vi "Start Sync.vi"(8 "error in (no error)":errorcluster, 10 "current time":timestamp, 11 "gRPC Server in":refnum<class "HVC5.lvclass">) -> (0 "error out":errorcluster, 3 "gRPC Server out":refnum<class "HVC5.lvclass">)   [LabVIEW 2019, in "HVC5.lvlib" / "HVC5.lvclass"]
uses:
  HVC5.lvclass
  RPC Messages/measurementservice_DMMConfigResponse/measurementservice_DMMConfigResponse_Data.ctl
  RPC Messages/measurementservice_ErrorOut/measurementservice_ErrorOut_Data.ctl
  RPC Messages/measurementservice_SMUConfigResponse/measurementservice_SMUConfigResponse_Data.ctl
  HVC5.lvclass/HVC5.ctl
  RPC Messages/measurementservice_QueryResponse/measurementservice_QueryResponse_Data.ctl
  RPC Messages/measurementservice_DMMOpenSessionResponse/measurementservice_DMMOpenSessionResponse_Data.ctl
  RPC Messages/measurementservice_DMMVoltageData/measurementservice_DMMVoltageData_Data.ctl
  RPC Messages/measurementservice_DMMCloseSessionResponse/measurementservice_DMMCloseSessionResponse_Data.ctl
  RPC Messages/measurementservice_DMMSelfCalResponse/measurementservice_DMMSelfCalResponse_Data.ctl
  RPC Messages/measurementservice_DMMResetResponse/measurementservice_DMMResetResponse_Data.ctl
  RPC Messages/measurementservice_SMUOpenSessionResponse/measurementservice_SMUOpenSessionResponse_Data.ctl
  RPC Messages/measurementservice_SMUCurrentData/measurementservice_SMUCurrentData_Data.ctl
  RPC Messages/measurementservice_SMUDisableResponse/measurementservice_SMUDisableResponse_Data.ctl
  RPC Messages/measurementservice_SMUEnableResponse/measurementservice_SMUEnableResponse_Data.ctl
  RPC Messages/measurementservice_SMUCloseSessionResponse/measurementservice_SMUCloseSessionResponse_Data.ctl
  RPC Messages/measurementservice_SMUSelfCalResponse/measurementservice_SMUSelfCalResponse_Data.ctl
  RPC Messages/measurementservice_SMUResetResponse/measurementservice_SMUResetResponse_Data.ctl
  RPC Messages/measurementservice_NI2576MUXOpenSessionResponse/measurementservice_NI2576MUXOpenSessionResponse_Data.ctl
  RPC Messages/measurementservice_NI2576MUXCloseSessionResponse/measurementservice_NI2576MUXCloseSessionResponse_Data.ctl
  RPC Messages/measurementservice_NI2576MUXDisconnectAllResponse/measurementservice_NI2576MUXDisconnectAllResponse_Data.ctl
  <instrlib>/niSwitch/niSwitch.llb/niSwitch Connect Channels (Single).vi
  RPC Messages/measurementservice_NI2576MUXCloseChannelResponse/measurementservice_NI2576MUXCloseChannelResponse_Data.ctl
  <instrlib>/niSwitch/niSwitch.llb/niSwitch Disconnect Channels (Single).vi
  RPC Messages/measurementservice_NI2576MUXOpenChannelResponse/measurementservice_NI2576MUXOpenChannelResponse_Data.ctl
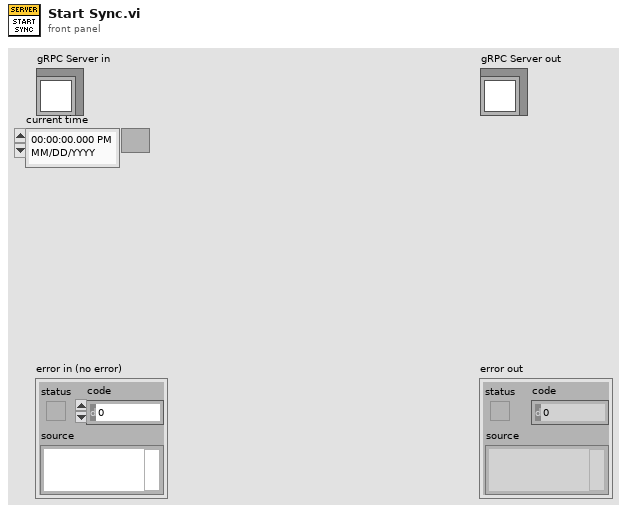
[diagram p1: front panel]
types:
  T1 = typedef "HVC5.lvlib/HVC5.lvclass/measurementservice_DMMConfigResponse_Data.ctl" = cluster{"DMMFunction":i32, "DMMResolution":sgl, "DMMRange":sgl, "DMMSampleCount":i32, "DMMApertureTimeUnit":i32, "DMMApertureTime":sgl, "DMMNumberofAverages":i32, "DMMAutoZero":i32, "DMMADCCalibration":i32, "DMMSettleTime":sgl, "error":T2}
  T2 = typedef "HVC5.lvlib/HVC5.lvclass/measurementservice_ErrorOut_Data.ctl" = cluster{"errCode":i32, "errMessage":string}
  T3 = typedef "HVC5.lvlib/HVC5.lvclass/measurementservice_SMUConfigResponse_Data.ctl" = cluster{"SMUChannels":string, "SMUSourceMode":i32, "SMUOutputFunction":i32, "SMUSourceTransientResponse":i32, "SMUCurrent":sgl, "SMUCurrentLevelRange":sgl, "SMUMeasurementSense":i32, "SMUApertureTimeUnit":i32, "SMUMeasurementApertureTime":sgl, "SMUSourceAdvancedSourceDelay":sgl, "SMUVoltage":sgl, "SMUMeasurementAdvancedDCNoiseRejection":i32, "error":T2}
  T4 = cluster{"DMMSession":refnum<k15>, "measurementservice_DMMConfigResponse_Data":T1, "SMUSession":refnum<k15>, "measurementservice_SMUConfigResponse_Data":T3, "NI2576Session":refnum<k15>}
  T5 = typedef "HVC5.lvlib/HVC5.lvclass/measurementservice_QueryResponse_Data.ctl" = cluster{"message":string, "status":i32}
  T6 = typedef "HVC5.lvlib/HVC5.lvclass/measurementservice_DMMOpenSessionResponse_Data.ctl" = cluster{"error":T2}
  T7 = typedef "HVC5.lvlib/HVC5.lvclass/measurementservice_DMMVoltageData_Data.ctl" = cluster{"voltage":sgl[], "error":T2}
  T8 = typedef "HVC5.lvlib/HVC5.lvclass/measurementservice_DMMCloseSessionResponse_Data.ctl" = cluster{"error":T2}
  T9 = typedef "HVC5.lvlib/HVC5.lvclass/measurementservice_DMMSelfCalResponse_Data.ctl" = cluster{"error":T2}
  T10 = typedef "HVC5.lvlib/HVC5.lvclass/measurementservice_DMMResetResponse_Data.ctl" = cluster{"error":T2}
  T11 = typedef "HVC5.lvlib/HVC5.lvclass/measurementservice_SMUOpenSessionResponse_Data.ctl" = cluster{"error":T2}
  T12 = typedef "HVC5.lvlib/HVC5.lvclass/measurementservice_SMUCurrentData_Data.ctl" = cluster{"current":sgl, "error":T2}
  T13 = typedef "HVC5.lvlib/HVC5.lvclass/measurementservice_SMUDisableResponse_Data.ctl" = cluster{"error":T2}
  T14 = typedef "HVC5.lvlib/HVC5.lvclass/measurementservice_SMUEnableResponse_Data.ctl" = cluster{"error":T2}
  T15 = typedef "HVC5.lvlib/HVC5.lvclass/measurementservice_SMUCloseSessionResponse_Data.ctl" = cluster{"error":T2}
  T16 = typedef "HVC5.lvlib/HVC5.lvclass/measurementservice_SMUSelfCalResponse_Data.ctl" = cluster{"error":T2}
  T17 = typedef "HVC5.lvlib/HVC5.lvclass/measurementservice_SMUResetResponse_Data.ctl" = cluster{"error":T2}
  T18 = typedef "HVC5.lvlib/HVC5.lvclass/measurementservice_NI2576MUXOpenSessionResponse_Data.ctl" = cluster{"error":T2}
  T19 = typedef "HVC5.lvlib/HVC5.lvclass/measurementservice_NI2576MUXCloseChannelResponse_Data.ctl" = cluster{"error":T2}
  T20 = typedef "HVC5.lvlib/HVC5.lvclass/measurementservice_NI2576MUXOpenChannelResponse_Data.ctl" = cluster{"error":T2}
  T21 = typedef "HVC5.lvlib/HVC5.lvclass/measurementservice_NI2576MUXDisconnectAllResponse_Data.ctl" = cluster{"error":T2}
  T22 = typedef "HVC5.lvlib/HVC5.lvclass/measurementservice_NI2576MUXCloseSessionResponse_Data.ctl" = cluster{"error":T2}
  T23 = typedef "HVC5.lvlib/HVC5.lvclass/Server gRPC UEs.ctl" = cluster{"Invoke gRPC UE":refnum<user-event>, "Query gRPC UE":refnum<user-event>, "Register gRPC UE":refnum<user-event>, "OpenDMMSession gRPC UE":refnum<user-event>, "ConfigureDMM gRPC UE":refnum<user-event>, "PerformDMMVoltageMeasurement gRPC UE":refnum<user-event>, "CloseDMMSession gRPC UE":refnum<user-event>, "SelfCalibrateDMM gRPC UE":refnum<user-event>, "ResetDMM gRPC UE":refnum<user-event>, "OpenSMUSession gRPC UE":refnum<user-event>, "ConfigureSMU gRPC UE":refnum<user-event>, "EnableSMUOutput gRPC UE":refnum<user-event>, "DisableSMUOutput gRPC UE":refnum<user-event>, "PerformSMUCurrentMeasurement gRPC UE":refnum<user-event>, "CloseSMUSession gRPC UE":refnum<user-event>, "SelfCalibrateSMU gRPC UE":refnum<user-event>, "ResetSMU gRPC UE":refnum<user-event>, "OpenNI2576MUXSession gRPC UE":refnum<user-event>, "CloseNI2576MUXChannel gRPC UE":refnum<user-event>, "OpenNI2576MUXChannel gRPC UE":refnum<user-event>, "DisconnectAllNI2576MUXChannels gRPC UE":refnum<user-event>, "CloseNI2576MUXSession gRPC UE":refnum<user-event>, "ResetNI2576MUX gRPC UE":refnum<user-event>}
  T24 = typedef "HVC5.lvlib/gprc-lvsupport.lvlib/grpcId.ctl" = u64
  T25 = typedef "HVC5.lvlib/HVC5.lvclass/measurementservice_QueryRequest_Data.ctl" = cluster{"query":string}
  T26 = typedef "HVC5.lvlib/HVC5.lvclass/measurementservice_DMMOpenSessionRequest_Data.ctl" = cluster{"DMMName":string}
  T27 = typedef "HVC5.lvlib/HVC5.lvclass/measurementservice_DMMConfigRequest_Data.ctl" = cluster{"DMMFunction":i32, "DMMResolution":sgl, "DMMRange":sgl, "DMMSampleCount":i32, "DMMApertureTimeUnit":i32, "DMMApertureTime":sgl, "DMMNumberofAverages":i32, "DMMAutoZero":i32, "DMMADCCalibration":i32, "DMMSettleTime":sgl}
  T28 = typedef "HVC5.lvlib/HVC5.lvclass/measurementservice_SMUOpenSessionRequest_Data.ctl" = cluster{"SMUName":string}
  T29 = typedef "HVC5.lvlib/HVC5.lvclass/measurementservice_SMUConfigRequest_Data.ctl" = cluster{"SMUChannels":string, "SMUSourceMode":i32, "SMUOutputFunction":i32, "SMUSourceTransientResponse":i32, "SMUCurrent":sgl, "SMUCurrentLevelRange":sgl, "SMUMeasurementSense":i32, "SMUApertureTimeUnit":i32, "SMUMeasurementApertureTime":sgl, "SMUSourceAdvancedSourceDelay":sgl, "SMUVoltage":sgl, "SMUMeasurementAdvancedDCNoiseRejection":i32}
  T30 = typedef "HVC5.lvlib/HVC5.lvclass/measurementservice_NI2576MUXOpenSessionRequest_Data.ctl" = cluster{"NI2576MUXName":string, "NI2576MUXTopology":string}
  T31 = typedef "HVC5.lvlib/HVC5.lvclass/measurementservice_NI2576MUXCloseChannelRequest_Data.ctl" = cluster{"Channel1":string, "Channel2":string}
  T32 = typedef "HVC5.lvlib/HVC5.lvclass/measurementservice_NI2576MUXOpenChannelRequest_Data.ctl" = cluster{"Channel1":string, "Channel2":string}
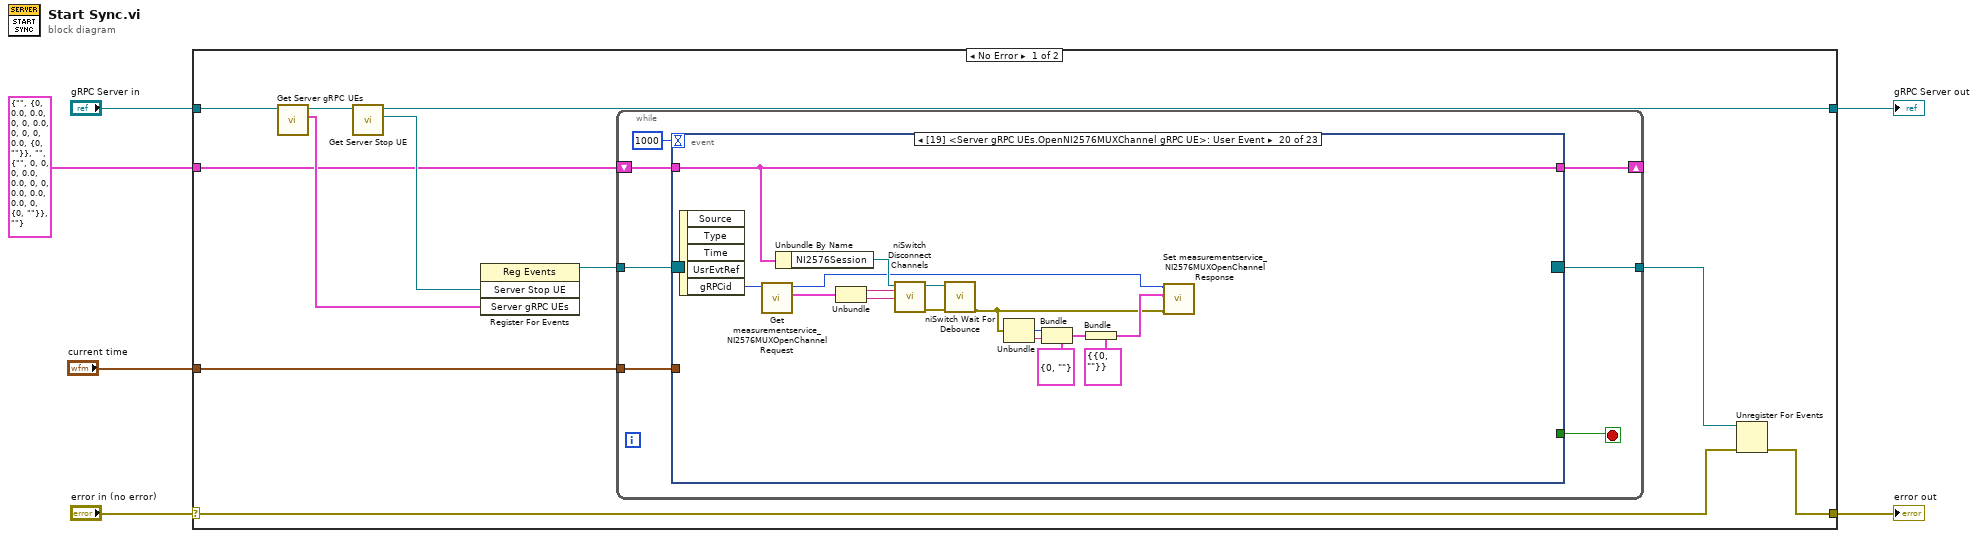
[diagram p0: block diagram]
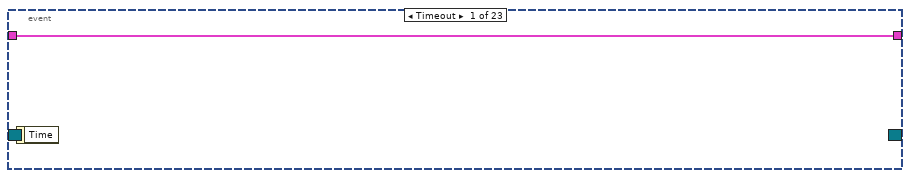
[diagram p2: hidden frame]
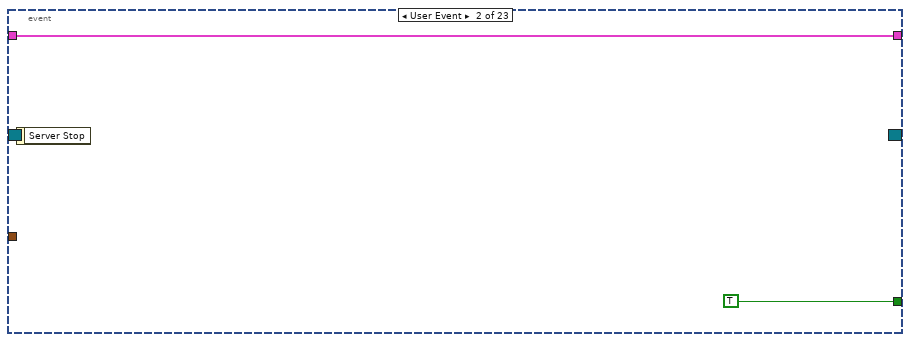
[diagram p3: hidden frame]
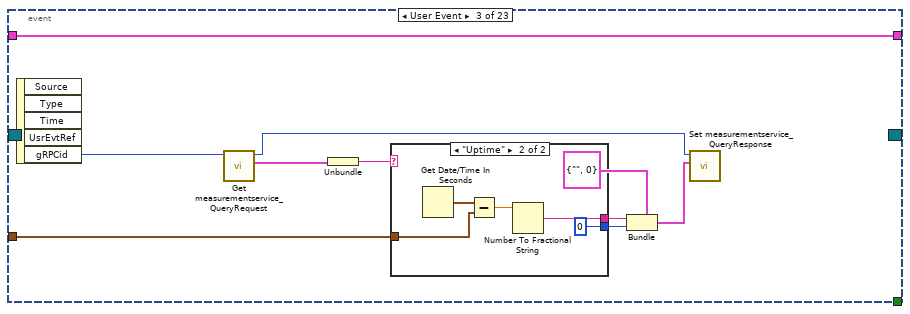
[diagram p4: hidden frame]
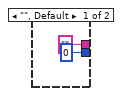
[diagram p5: hidden frame]
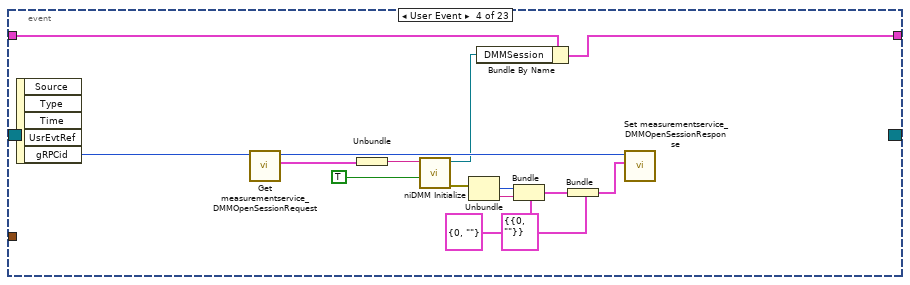
[diagram p6: hidden frame]
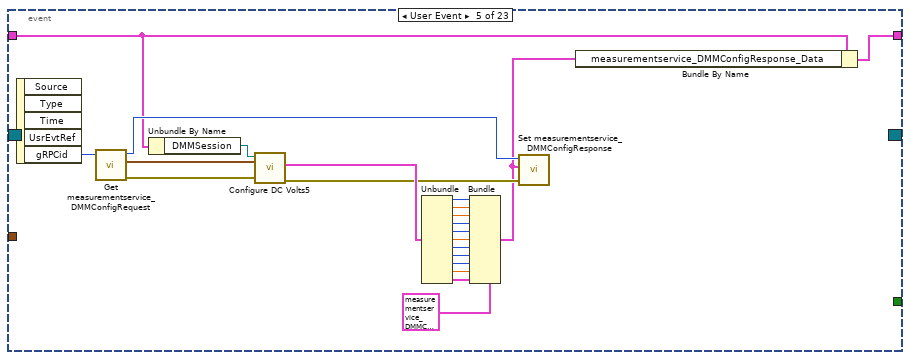
[diagram p7: hidden frame]
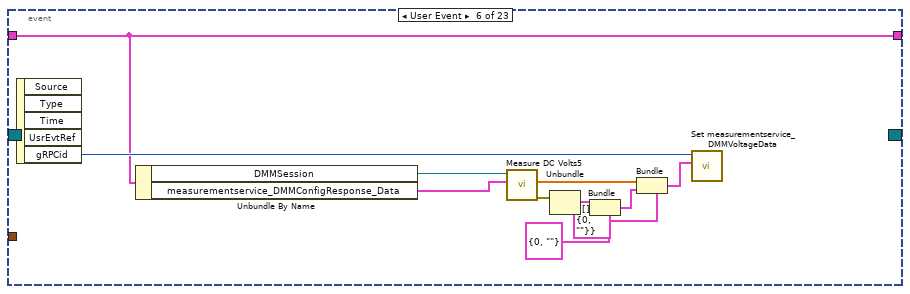
[diagram p8: hidden frame]
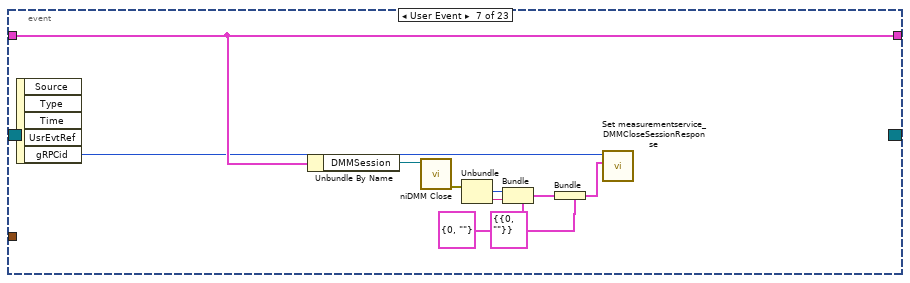
[diagram p9: hidden frame]
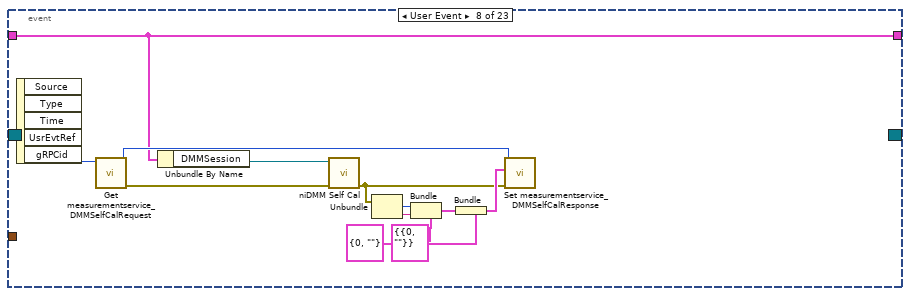
[diagram p10: hidden frame]
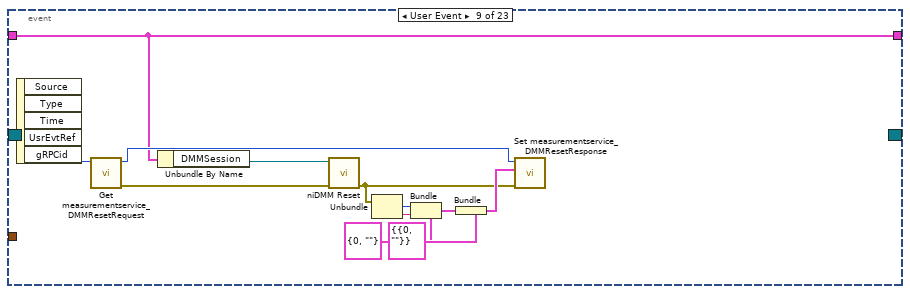
[diagram p11: hidden frame]
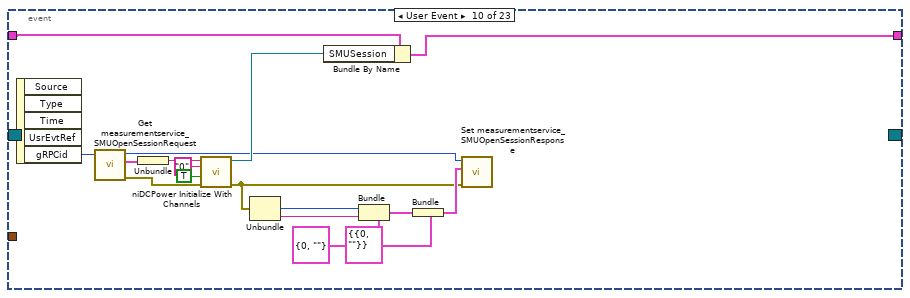
[diagram p12: hidden frame]
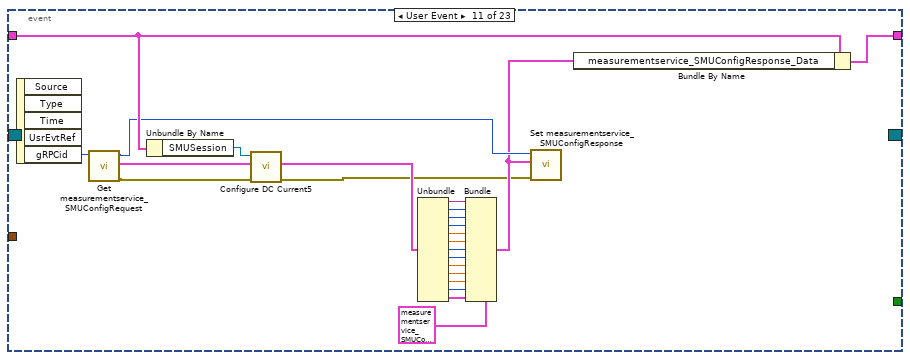
[diagram p13: hidden frame]
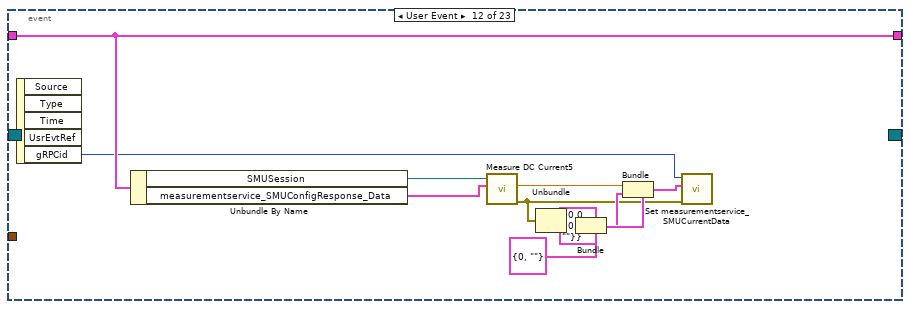
[diagram p14: hidden frame]
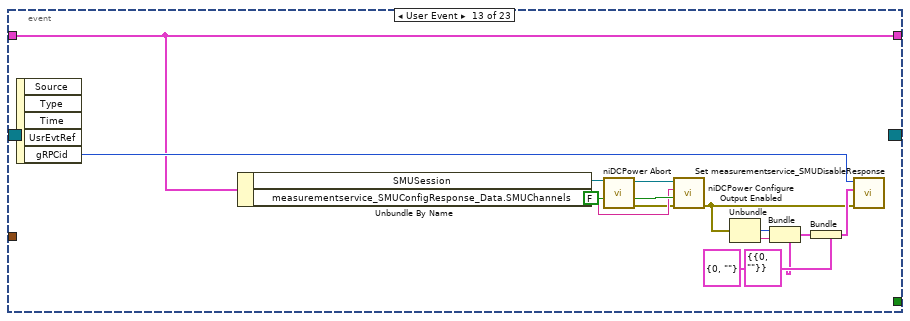
[diagram p15: hidden frame]
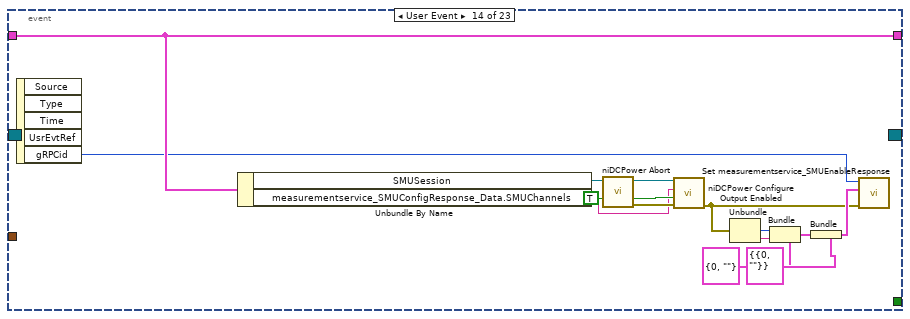
[diagram p16: hidden frame]
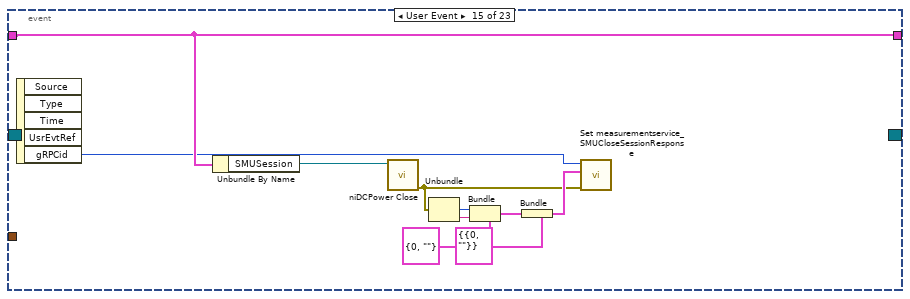
[diagram p17: hidden frame]
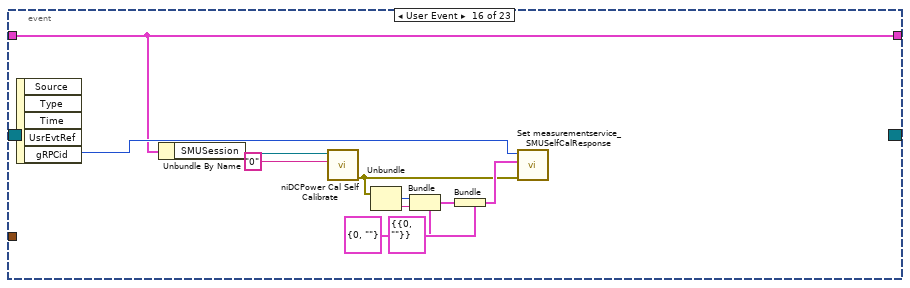
[diagram p18: hidden frame]
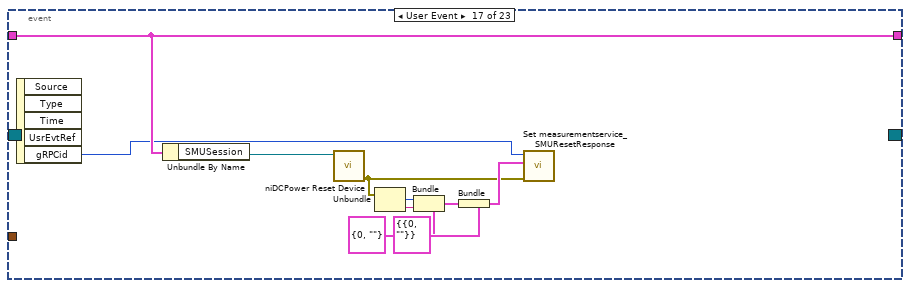
[diagram p19: hidden frame]
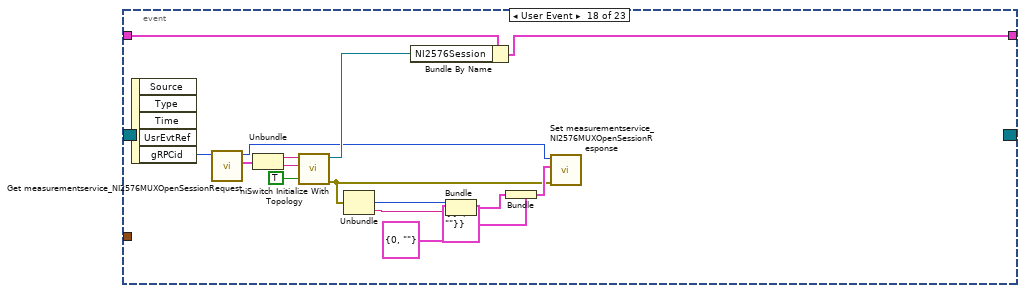
[diagram p20: hidden frame]
diagram:
  n1 = case shown="No Error" "error in (no error)" {
    selector: "error in (no error)" -> [w10 w318]
    tunnel: [w9 w318] -> w5
    tunnel: [w13 w317] -> w3
    tunnel: "gRPC Server in" -> [w17 w317]
    tunnel: "current time" -> [w8 _]
    tunnel: T4 {"DMMSession"="", "measurementservice_DMMConfigResponse_Data"={"DMMFunction"=0, "DMMResolution"=0.0, "DMMRange"=0.0, "DMMSampleCount"=0, "DMMApertureTimeUnit"=0, "DMMApertureTime"=0.0, "DMMNumberofAverages"=0, "DMMAutoZero"=0, "DMMADCCalibration"=0, "DMMSettleTime"=0.0, "error"={"errCode"=0, "errMessage"=""}}, "SMUSession"="", "measurementservice_SMUConfigResponse_Data"={"SMUChannels"="", "SMUSourceMode"=0, "SMUOutputFunction"=0, "SMUSourceTransientResponse"=0, "SMUCurrent"=0.0, "SMUCurrentLevelRange"=0.0, "SMUMeasurementSense"=0, "SMUApertureTimeUnit"=0, "SMUMeasurementApertureTime"=0.0, "SMUSourceAdvancedSourceDelay"=0.0, "SMUVoltage"=0.0, "SMUMeasurementAdvancedDCNoiseRejection"=0, "error"={"errCode"=0, "errMessage"=""}}, "NI2576Session"=""} -> [w7 _]
    frame No Error {
      n2 = call "Get Server gRPC UEs.vi"("OOP Server in"=w17) -> ("Server gRPC UEs"=w14:T23, "OOP Server out"=w16:refnum<class "HVC5.lvclass">)  [unwired: 9 in]
      n3 = call "Get Server Stop UE.vi"("OOP Server in"=w16) -> ("Server Stop UE"=w15:refnum<user-event>, "OOP Server out"=w13:refnum<class "HVC5.lvclass">)  [unwired: 9 in]
      n4 = register-events(w15, w14) -> (reference out=w12:refnum<event-registration>)  [unwired: 2 in, 1 out]
      n5 = while {
        tunnel: w12 -> [w24]
        tunnel: [w22] -> w11
        tunnel: w8 -> [w20]
        shift-right: [w18] -> _
        shift-left: w7 -> [w19]
        stop <- w23 stop-if-true
        n6 = event "RPC Methods Event Structure" shown="[19] <Server gRPC UEs.OpenNI2576MUXChannel gRPC UE>: User Event" {
          selector: w24 -> [_ _ _ _ _ _ _ _ _ _ _ _ _ _ _ _ _ _ _ _ _ _ _]
          dyn-events: [_ _ _ _ _ _ _ _ _ _ _ _ _ _ _ _ _ _ _ _ _ _ _] -> w22
          timeout: 1000 -> [_ _ _ _ _ _ _ _ _ _ _ _ _ _ _ _ _ _ _ _ _ _ _]
          tunnel: [_ TRUE _ _ _ _ _ _ _ _ _ _ _ _ _ _ _ _ _ _ _ _ _] -> w23
          tunnel: w20 -> [_ _ w35 _ _ _ _ _ _ _ _ _ _ _ _ _ _ _ _ _ _ _ _]
          tunnel: w19 -> [w25 w26 w28 w47 w62 w82 w96 w104 w116 w137 w157 w178 w185 w205 w215 w219 w237 w250 w264 w282 w288 w298 w308]
          tunnel: [w25 w26 w28 w45 w60 w82 w96 w104 w116 w136 w156 w178 w185 w205 w215 w219 w237 w248 w264 w282 w288 w298 w308] -> w18
          event Timeout {
            n7 = event-data() -> ()  [unwired: 1 in, 1 out]
          }
          event User Event {
            n8 = event-data() -> ()  [unwired: 1 in, 1 out]
          }
          event User Event {
            n9 = event-data() -> ("gRPCid"=w37:T24)  [unwired: 1 in, 4 out]
            n10 = call "Get measurementservice_QueryRequest.vi"("gRPCid"=w37) -> ("Message Data"=w36:T25, "gRPCid out"=w30:T24)  [unwired: 8 in, 1 out]
            n11 = Unbundle(w36) -> ("query"=w34:string)
            n12 = case shown="\"Uptime\"" w34 {
              tunnel: w35 -> [_ w43]
              tunnel: ["" w41] -> w32
              tunnel: [0 ("status") 0 ("status")] -> w31
              frame "", Default {
              }
              frame "Uptime" {
                n13 = Get Date/Time In Seconds() -> (seconds since 1Jan1904=w44:timestamp)
                n14 = Subtract(x=w44, y=w43) -> (x-y=w42:dbl)
                n15 = Number To Fractional String(number=w42) -> (F-format string=w41:string)  [unwired: 3 in]
              }
            }
            n16 = Bundle(cluster=T5 {"message"="", "status"=0} ("measurementservice_QueryResponse_Data"), "message"=w32, "status"=w31) -> (w29:T5)
            n17 = call "Set measurementservice_QueryResponse.vi"("Message Data"=w29, "gRPCid"=w30) -> ()  [unwired: 9 in, 1 out]
          }
          event User Event {
            n18 = event-data() -> ("gRPCid"=w59:T24)  [unwired: 1 in, 4 out]
            n19 = call "Get measurementservice_DMMOpenSessionRequest.vi"("gRPCid"=w59) -> ("Message Data"=w58:T26, "gRPCid out"=w48:T24)  [unwired: 8 in, 1 out]
            n20 = Unbundle(w58) -> ("DMMName"=w57:string)
            n21 = call <instrlib>:"niDMM Initialize.vi"("Reset"=TRUE, "Instrument Descriptor"=w57) -> ("error out"=w55:errorcluster, "instrument handle out"=w46:refnum<k15>)  [unwired: 8 in]
            n22 = Unbundle(w55) -> ("code"=w52:i32, "source"=w51:string)  [unwired: 1 out]
            n23 = Bundle By Name(cluster=w47, "DMMSession"=w46) -> (w45:T4)
            n24 = Bundle(cluster=T2 {"errCode"=0, "errMessage"=""} ("error"), "errCode"=w52, "errMessage"=w51) -> (w50:T2)
            n25 = Bundle(cluster=T6 {"error"={"errCode"=0, "errMessage"=""}} ("measurementservice_DMMOpenSessionResponse_Data"), "error"=w50) -> (w49:T6)
            n26 = call "Set measurementservice_DMMOpenSessionResponse.vi"("Message Data"=w49, "gRPCid"=w48) -> ()  [unwired: 9 in, 1 out]
          }
          event User Event {
            n27 = event-data() -> ("gRPCid"=w81:T24)  [unwired: 1 in, 4 out]
            n28 = call "Get measurementservice_DMMConfigRequest.vi"("gRPCid"=w81) -> ("error out"=w65:errorcluster, "Message Data"=w80:T27, "gRPCid out"=w77:T24)  [unwired: 8 in]
            n29 = Unbundle By Name(w62) -> ("DMMSession"=w79:refnum<k15>)
            n30 = call "Configure DC Volts5.vi"("error in (no error)"=w65, "measurementservice_DMMConfigRequest_Data"=w80, "DMMSession"=w79) -> ("error out"=w63:errorcluster, "measurementservice_DMMConfigResponse_Data"=w76:T1)  [unwired: 7 in]
            n31 = Unbundle(w76) -> ("DMMFunction"=w75:i32, "DMMResolution"=w74:sgl, "DMMRange"=w73:sgl, "DMMSampleCount"=w72:i32, "DMMApertureTimeUnit"=w71:i32, "DMMApertureTime"=w70:sgl, "DMMNumberofAverages"=w69:i32, "DMMAutoZero"=w68:i32, "DMMADCCalibration"=w67:i32, "DMMSettleTime"=w66:sgl, "error"=w64:T2)
            n32 = Bundle(cluster=T1 {"DMMFunction"=0, "DMMResolution"=0.0, "DMMRange"=0.0, "DMMSampleCount"=0, "DMMApertureTimeUnit"=0, "DMMApertureTime"=0.0, "DMMNumberofAverages"=0, "DMMAutoZero"=0, "DMMADCCalibration"=0, "DMMSettleTime"=0.0, "error"={"errCode"=0, "errMessage"=""}} ("measurementservice_DMMConfigResponse_Data"), "DMMFunction"=w75, "DMMResolution"=w74, "DMMRange"=w73, "DMMSampleCount"=w72, "DMMApertureTimeUnit"=w71, "DMMApertureTime"=w70, "DMMNumberofAverages"=w69, "DMMAutoZero"=w68, "DMMADCCalibration"=w67, "DMMSettleTime"=w66, "error"=w64) -> (w61:T1)
            n33 = call "Set measurementservice_DMMConfigResponse.vi"("error in (no error)"=w63, "Message Data"=w61, "gRPCid"=w77) -> ()  [unwired: 8 in, 1 out]
            n34 = Bundle By Name(cluster=w62, "measurementservice_DMMConfigResponse_Data"=w61) -> (w60:T4)
          }
          event User Event {
            n35 = event-data() -> ("gRPCid"=w83:T24)  [unwired: 1 in, 4 out]
            n36 = Unbundle By Name(w82) -> ("DMMSession"=w93:refnum<k15>, "measurementservice_DMMConfigResponse_Data"=w92:T1)
            n37 = call "Measure DC Volts5.vi"("measurementservice_DMMConfigResponse_Data"=w92, "DMMSession"=w93) -> ("error out"=w88:errorcluster, "Measurement Array (Volts)"=w90:sgl[])  [unwired: 8 in]
            n38 = Unbundle(w88) -> ("code"=w87:i32, "source"=w86:string)  [unwired: 1 out]
            n39 = Bundle(cluster=T2 {"errCode"=0, "errMessage"=""} ("error"), "errCode"=w87, "errMessage"=w86) -> (w85:T2)
            n40 = Bundle(cluster=T7 {"voltage"=[], "error"={"errCode"=0, "errMessage"=""}} ("Message Data"), "voltage"=w90, "error"=w85) -> (w84:T7)
            n41 = call "Set measurementservice_DMMVoltageData.vi"("Message Data"=w84, "gRPCid"=w83) -> ()  [unwired: 9 in, 1 out]
          }
          event User Event {
            n42 = event-data() -> ("gRPCid"=w94:T24)  [unwired: 1 in, 4 out]
            n43 = Unbundle By Name(w96) -> ("DMMSession"=w95:refnum<k15>)
            n44 = call <instrlib>:"niDMM Close.vi"("instrument handle"=w95) -> ("error out"=w103:errorcluster)  [unwired: 10 in]
            n45 = Unbundle(w103) -> ("code"=w99:i32, "source"=w98:string)  [unwired: 1 out]
            n46 = Bundle(cluster=T2 {"errCode"=0, "errMessage"=""} ("error"), "errCode"=w99, "errMessage"=w98) -> (w97:T2)
            n47 = Bundle(cluster=T8 {"error"={"errCode"=0, "errMessage"=""}} ("measurementservice_DMMCloseSessionResponse_Data"), "error"=w97) -> (w101:T8)
            n48 = call "Set measurementservice_DMMCloseSessionResponse.vi"("Message Data"=w101, "gRPCid"=w94) -> ()  [unwired: 9 in, 1 out]
          }
          event User Event {
            n49 = event-data() -> ("gRPCid"=w115:T24)  [unwired: 1 in, 4 out]
            n50 = call "Get measurementservice_DMMSelfCalRequest.vi"("gRPCid"=w115) -> ("error out"=w106:errorcluster, "gRPCid out"=w108:T24)  [unwired: 8 in, 1 out]
            n51 = Unbundle By Name(w104) -> ("DMMSession"=w105:refnum<k15>)
            n52 = call <instrlib>:"niDMM Self Cal.vi"("error in (no error)"=w106, "instrument handle"=w105) -> ("error out"=w107:errorcluster)  [unwired: 8 in, 1 out]
            n53 = Unbundle(w107) -> ("code"=w110:i32, "source"=w109:string)  [unwired: 1 out]
            n54 = Bundle(cluster=T2 {"errCode"=0, "errMessage"=""} ("error"), "errCode"=w110, "errMessage"=w109) -> (w111:T2)
            n55 = Bundle(cluster=T9 {"error"={"errCode"=0, "errMessage"=""}} ("measurementservice_DMMSelfCalResponse_Data"), "error"=w111) -> (w113:T9)
            n56 = call "Set measurementservice_DMMSelfCalResponse.vi"("error in (no error)"=w107, "Message Data"=w113, "gRPCid"=w108) -> ()  [unwired: 8 in, 1 out]
          }
          event User Event {
            n57 = event-data() -> ("gRPCid"=w124:T24)  [unwired: 1 in, 4 out]
            n58 = call "Get measurementservice_DMMResetRequest.vi"("gRPCid"=w124) -> ("error out"=w123:errorcluster, "gRPCid out"=w120:T24)  [unwired: 8 in, 1 out]
            n59 = Unbundle By Name(w116) -> ("DMMSession"=w125:refnum<k15>)
            n60 = call <instrlib>:"niDMM Reset.vi"("error in (no error)"=w123, "instrument handle"=w125) -> ("error out"=w119:errorcluster)  [unwired: 8 in, 1 out]
            n61 = Unbundle(w119) -> ("code"=w127:i32, "source"=w126:string)  [unwired: 1 out]
            n62 = Bundle(cluster=T2 {"errCode"=0, "errMessage"=""} ("error"), "errCode"=w127, "errMessage"=w126) -> (w117:T2)
            n63 = Bundle(cluster=T10 {"error"={"errCode"=0, "errMessage"=""}} ("measurementservice_DMMResetResponse_Data"), "error"=w117) -> (w121:T10)
            n64 = call "Set measurementservice_DMMResetResponse.vi"("error in (no error)"=w119, "Message Data"=w121, "gRPCid"=w120) -> ()  [unwired: 8 in, 1 out]
          }
          event User Event {
            n65 = event-data() -> ("gRPCid"=w139:T24)  [unwired: 1 in, 4 out]
            n66 = call "Get measurementservice_SMUOpenSessionRequest.vi"("gRPCid"=w139) -> ("error out"=w130:errorcluster, "Message Data"=w138:T28, "gRPCid out"=w135:T24)  [unwired: 8 in]
            n67 = Unbundle(w138) -> ("SMUName"=w144:string)
            n68 = call <instrlib>:"niDCPower Initialize With Channels.vi"("error in (no error)"=w130, "reset (false)"=TRUE ("Reset"), "channels"="0", "resource name"=w144) -> ("error out"=w129:errorcluster, "instrument handle out"=w140:refnum<k15>)  [unwired: 6 in]
            n69 = Unbundle(w129) -> ("code"=w142:i32, "source"=w141:string)  [unwired: 1 out]
            n70 = Bundle By Name(cluster=w137, "SMUSession"=w140) -> (w136:T4)
            n71 = Bundle(cluster=T2 {"errCode"=0, "errMessage"=""} ("error"), "errCode"=w142, "errMessage"=w141) -> (w131:T2)
            n72 = Bundle(cluster=T11 {"error"={"errCode"=0, "errMessage"=""}} ("measurementservice_SMUOpenSessionResponse_Data"), "error"=w131) -> (w134:T11)
            n73 = call "Set measurementservice_SMUOpenSessionResponse.vi"("error in (no error)"=w129, "Message Data"=w134, "gRPCid"=w135) -> ()  [unwired: 8 in, 1 out]
          }
          event User Event {
            n74 = event-data() -> ("gRPCid"=w155:T24)  [unwired: 1 in, 4 out]
            n75 = call "Get measurementservice_SMUConfigRequest.vi"("gRPCid"=w155) -> ("error out"=w154:errorcluster, "Message Data"=w152:T29, "gRPCid out"=w150:T24)  [unwired: 8 in]
            n76 = Unbundle By Name(w157) -> ("SMUSession"=w153:refnum<k15>)
            n77 = call "Configure DC Current5.vi"("error in (no error)"=w154, "measurementservice_SMUConfigRequest_Data"=w152, "SMUSession"=w153) -> ("error out"=w145:errorcluster, "measurementservice_SMUConfigResponse_Data"=w151:T3)  [unwired: 7 in]
            n78 = Unbundle(w151) -> ("SMUChannels"=w168:string, "SMUSourceMode"=w167:i32, "SMUOutputFunction"=w166:i32, "SMUSourceTransientResponse"=w165:i32, "SMUCurrent"=w164:sgl, "SMUCurrentLevelRange"=w163:sgl, "SMUMeasurementSense"=w162:i32, "SMUApertureTimeUnit"=w161:i32, "SMUMeasurementApertureTime"=w160:sgl, "SMUSourceAdvancedSourceDelay"=w159:sgl, "SMUVoltage"=w158:sgl, "SMUMeasurementAdvancedDCNoiseRejection"=w147:i32, "error"=w148:T2)
            n79 = Bundle(cluster=T3 {"SMUChannels"="", "SMUSourceMode"=0, "SMUOutputFunction"=0, "SMUSourceTransientResponse"=0, "SMUCurrent"=0.0, "SMUCurrentLevelRange"=0.0, "SMUMeasurementSense"=0, "SMUApertureTimeUnit"=0, "SMUMeasurementApertureTime"=0.0, "SMUSourceAdvancedSourceDelay"=0.0, "SMUVoltage"=0.0, "SMUMeasurementAdvancedDCNoiseRejection"=0, "error"={"errCode"=0, "errMessage"=""}} ("Message Data"), "SMUChannels"=w168, "SMUSourceMode"=w167, "SMUOutputFunction"=w166, "SMUSourceTransientResponse"=w165, "SMUCurrent"=w164, "SMUCurrentLevelRange"=w163, "SMUMeasurementSense"=w162, "SMUApertureTimeUnit"=w161, "SMUMeasurementApertureTime"=w160, "SMUSourceAdvancedSourceDelay"=w159, "SMUVoltage"=w158, "SMUMeasurementAdvancedDCNoiseRejection"=w147, "error"=w148) -> (w146:T3)
            n80 = call "Set measurementservice_SMUConfigResponse.vi"("error in (no error)"=w145, "Message Data"=w146, "gRPCid"=w150) -> ()  [unwired: 8 in, 1 out]
            n81 = Bundle By Name(cluster=w157, "measurementservice_SMUConfigResponse_Data"=w146) -> (w156:T4)
          }
          event User Event {
            n82 = event-data() -> ("gRPCid"=w173:T24)  [unwired: 1 in, 4 out]
            n83 = Unbundle By Name(w178) -> ("SMUSession"=w177:refnum<k15>, "measurementservice_SMUConfigResponse_Data"=w176:T3)
            n84 = call "Measure DC Current5.vi"("measurementservice_SMUConfigResponse_Data"=w176, "SMUSession"=w177) -> ("error out"=w169:errorcluster, "Current Measurement"=w175:sgl)  [unwired: 6 in, 2 out]
            n85 = Unbundle(w169) -> ("code"=w180:i32, "source"=w179:string)  [unwired: 1 out]
            n86 = Bundle(cluster=T2 {"errCode"=0, "errMessage"=""} ("error"), "errCode"=w180, "errMessage"=w179) -> (w170:T2)
            n87 = Bundle(cluster=T12 {"current"=0.0, "error"={"errCode"=0, "errMessage"=""}} ("measurementservice_SMUCurrentData_Data"), "current"=w175, "error"=w170) -> (w172:T12)
            n88 = call "Set measurementservice_SMUCurrentData.vi"("error in (no error)"=w169, "Message Data"=w172, "gRPCid"=w173) -> ()  [unwired: 8 in, 1 out]
          }
          event User Event {
            n89 = event-data() -> ("gRPCid"=w187:T24)  [unwired: 1 in, 4 out]
            n90 = Unbundle By Name(w185) -> ("SMUSession"=w184:refnum<k15>, "measurementservice_SMUConfigResponse_Data.SMUChannels"=w182:string)
            n91 = call <instrlib>:"niDCPower Abort.vi"("instrument handle"=w184) -> ("error out"=w181:errorcluster, "instrument handle out"=w183:refnum<k15>)  [unwired: 9 in]
            n92 = call <instrlib>:"niDCPower Configure Output Enabled.vi"("error in (no error)"=w181, "output enabled"=FALSE, "channel name"=w182, "instrument handle"=w183) -> ("error out"=w186:errorcluster)  [unwired: 6 in, 1 out]
            n93 = Unbundle(w186) -> ("code"=w189:i32, "source"=w188:string)  [unwired: 1 out]
            n94 = Bundle(cluster=T2 {"errCode"=0, "errMessage"=""} ("error"), "errCode"=w189, "errMessage"=w188) -> (w191:T2)
            n95 = Bundle(cluster=T13 {"error"={"errCode"=0, "errMessage"=""}} ("measurementservice_SMUDisableResponse_Data"), "error"=w191) -> (w190:T13)
            n96 = call "Set measurementservice_SMUDisableResponse.vi"("error in (no error)"=w186, "Message Data"=w190, "gRPCid"=w187) -> ()  [unwired: 8 in, 1 out]
          }
          event User Event {
            n97 = event-data() -> ("gRPCid"=w203:T24)  [unwired: 1 in, 4 out]
            n98 = Unbundle By Name(w205) -> ("SMUSession"=w198:refnum<k15>, "measurementservice_SMUConfigResponse_Data.SMUChannels"=w195:string)
            n99 = call <instrlib>:"niDCPower Abort.vi"("instrument handle"=w198) -> ("error out"=w197:errorcluster, "instrument handle out"=w196:refnum<k15>)  [unwired: 9 in]
            n100 = call <instrlib>:"niDCPower Configure Output Enabled.vi"("error in (no error)"=w197, "output enabled"=TRUE, "channel name"=w195, "instrument handle"=w196) -> ("error out"=w201:errorcluster)  [unwired: 6 in, 1 out]
            n101 = Unbundle(w201) -> ("code"=w207:i32, "source"=w206:string)  [unwired: 1 out]
            n102 = Bundle(cluster=T2 {"errCode"=0, "errMessage"=""} ("error"), "errCode"=w207, "errMessage"=w206) -> (w199:T2)
            n103 = Bundle(cluster=T14 {"error"={"errCode"=0, "errMessage"=""}} ("measurementservice_SMUEnableResponse_Data"), "error"=w199) -> (w202:T14)
            n104 = call "Set measurementservice_SMUEnableResponse.vi"("error in (no error)"=w201, "Message Data"=w202, "gRPCid"=w203) -> ()  [unwired: 8 in, 1 out]
          }
          event User Event {
            n105 = event-data() -> ("gRPCid"=w214:T24)  [unwired: 1 in, 4 out]
            n106 = Unbundle By Name(w215) -> ("SMUSession"=w216:refnum<k15>)
            n107 = call <instrlib>:"niDCPower Close.vi"("instrument handle"=w216) -> ("error out"=w209:errorcluster)  [unwired: 10 in]
            n108 = Unbundle(w209) -> ("code"=w218:i32, "source"=w217:string)  [unwired: 1 out]
            n109 = Bundle(cluster=T2 {"errCode"=0, "errMessage"=""} ("error"), "errCode"=w218, "errMessage"=w217) -> (w210:T2)
            n110 = Bundle(cluster=T15 {"error"={"errCode"=0, "errMessage"=""}} ("measurementservice_SMUCloseSessionResponse_Data"), "error"=w210) -> (w213:T15)
            n111 = call "Set measurementservice_SMUCloseSessionResponse.vi"("error in (no error)"=w209, "Message Data"=w213, "gRPCid"=w214) -> ()  [unwired: 8 in, 1 out]
          }
          event User Event {
            n112 = event-data() -> ("gRPCid"=w225:T24)  [unwired: 1 in, 4 out]
            n113 = Unbundle By Name(w219) -> ("SMUSession"=w227:refnum<k15>)
            n114 = call <instrlib>:"niDCPower Cal Self Calibrate.vi"("channel name"="0", "instrument handle"=w227) -> ("error out"=w223:errorcluster)  [unwired: 8 in, 1 out]
            n115 = Unbundle(w223) -> ("code"=w229:i32, "source"=w228:string)  [unwired: 1 out]
            n116 = Bundle(cluster=T2 {"errCode"=0, "errMessage"=""} ("error"), "errCode"=w229, "errMessage"=w228) -> (w220:T2)
            n117 = Bundle(cluster=T16 {"error"={"errCode"=0, "errMessage"=""}} ("measurementservice_SMUSelfCalResponse_Data"), "error"=w220) -> (w224:T16)
            n118 = call "Set measurementservice_SMUSelfCalResponse.vi"("error in (no error)"=w223, "Message Data"=w224, "gRPCid"=w225) -> ()  [unwired: 8 in, 1 out]
          }
          event User Event {
            n119 = event-data() -> ("gRPCid"=w230:T24)  [unwired: 1 in, 4 out]
            n120 = Unbundle By Name(w237) -> ("SMUSession"=w236:refnum<k15>)
            n121 = call <instrlib>:"niDCPower Reset Device.vi"("instrument handle"=w236) -> ("error out"=w234:errorcluster)  [unwired: 9 in, 1 out]
            n122 = Unbundle(w234) -> ("code"=w239:i32, "source"=w238:string)  [unwired: 1 out]
            n123 = Bundle(cluster=T2 {"errCode"=0, "errMessage"=""} ("error"), "errCode"=w239, "errMessage"=w238) -> (w231:T2)
            n124 = Bundle(cluster=T17 {"error"={"errCode"=0, "errMessage"=""}} ("measurementservice_SMUResetResponse_Data"), "error"=w231) -> (w235:T17)
            n125 = call "Set measurementservice_SMUResetResponse.vi"("error in (no error)"=w234, "Message Data"=w235, "gRPCid"=w230) -> ()  [unwired: 8 in, 1 out]
          }
          event User Event {
            n126 = event-data() -> ("gRPCid"=w255:T24)  [unwired: 1 in, 4 out]
            n127 = call "Get measurementservice_NI2576MUXOpenSessionRequest.vi"("gRPCid"=w255) -> ("Message Data"=w254:T30, "gRPCid out"=w245:T24)  [unwired: 8 in, 1 out]
            n128 = Unbundle(w254) -> ("NI2576MUXName"=w253:string, "NI2576MUXTopology"=w252:string)
            n129 = call <instrlib>:"niSwitch Initialize With Topology.vi"("reset device (boolean value)"=TRUE, "topology name"=w252, "resource name"=w253) -> ("error out"=w240:errorcluster, "instrument handle out"=w249:refnum<k15>)  [unwired: 7 in]
            n130 = Unbundle(w240) -> ("code"=w242:i32, "source"=w241:string)  [unwired: 1 out]
            n131 = Bundle By Name(cluster=w250, "NI2576Session"=w249) -> (w248:T4)
            n132 = Bundle(cluster=T2 {"errCode"=0, "errMessage"=""} ("error"), "errCode"=w242, "errMessage"=w241) -> (w243:T2)
            n133 = Bundle(cluster=T18 {"error"={"errCode"=0, "errMessage"=""}} ("measurementservice_NI2576MUXOpenSessionResponse_Data"), "error"=w243) -> (w246:T18)
            n134 = call "Set measurementservice_NI2576MUXOpenSessionResponse.vi"("error in (no error)"=w240, "Message Data"=w246, "gRPCid"=w245) -> ()  [unwired: 8 in, 1 out]
          }
          event User Event {
            n135 = event-data() -> ("gRPCid"=w269:T24)  [unwired: 1 in, 4 out]
            n136 = call "Get measurementservice_NI2576MUXCloseChannelRequest.vi"("gRPCid"=w269) -> ("Message Data"=w268:T31, "gRPCid out"=w263:T24)  [unwired: 8 in, 1 out]
            n137 = Unbundle By Name(w264) -> ("NI2576Session"=w267:refnum<k15>)
            n138 = Unbundle(w268) -> ("Channel1"=w266:string, "Channel2"=w265:string)
            n139 = call-poly <instrlib>:"niSwitch Connect Channels.vi"("channel 2"=w265, "channel 1"=w266, "instrument handle"=w267) -> ("error out"=w256:errorcluster, "instrument handle out"=w258:refnum<k15>)  [unwired: 7 in]
            n140 = call <instrlib>:"niSwitch Wait For Debounce.vi"("error in (no error)"=w256, "instrument handle"=w258) -> ("error out"=w257:errorcluster)  [unwired: 8 in, 1 out]
            n141 = Unbundle(w257) -> ("code"=w271:i32, "source"=w270:string)  [unwired: 1 out]
            n142 = Bundle(cluster=T2 {"errCode"=0, "errMessage"=""} ("error"), "errCode"=w271, "errMessage"=w270) -> (w259:T2)
            n143 = Bundle(cluster=T19 {"error"={"errCode"=0, "errMessage"=""}} ("measurementservice_NI2576MUXCloseChannelResponse_Data"), "error"=w259) -> (w262:T19)
            n144 = call "Set measurementservice_NI2576MUXCloseChannelResponse.vi"("error in (no error)"=w257, "Message Data"=w262, "gRPCid"=w263) -> ()  [unwired: 8 in, 1 out]
          }
          event User Event {
            n145 = event-data() -> ("gRPCid"=w279:T24)  [unwired: 1 in, 4 out]
            n146 = call "Get measurementservice_NI2576MUXOpenChannelRequest.vi"("gRPCid"=w279) -> ("Message Data"=w278:T32, "gRPCid out"=w277:T24)  [unwired: 8 in, 1 out]
            n147 = Unbundle By Name(w282) -> ("NI2576Session"=w285:refnum<k15>)
            n148 = Unbundle(w278) -> ("Channel1"=w284:string, "Channel2"=w283:string)
            n149 = call-poly <instrlib>:"niSwitch Disconnect Channels.vi"("channel 2"=w283, "channel 1"=w284, "instrument handle"=w285) -> ("error out"=w280:errorcluster, "instrument handle out"=w281:refnum<k15>)  [unwired: 7 in]
            n150 = call <instrlib>:"niSwitch Wait For Debounce.vi"("error in (no error)"=w280, "instrument handle"=w281) -> ("error out"=w275:errorcluster)  [unwired: 8 in, 1 out]
            n151 = Unbundle(w275) -> ("code"=w287:i32, "source"=w286:string)  [unwired: 1 out]
            n152 = Bundle(cluster=T2 {"errCode"=0, "errMessage"=""} ("error"), "errCode"=w287, "errMessage"=w286) -> (w272:T2)
            n153 = Bundle(cluster=T20 {"error"={"errCode"=0, "errMessage"=""}} ("measurementservice_NI2576MUXOpenChannelResponse_Data"), "error"=w272) -> (w276:T20)
            n154 = call "Set measurementservice_NI2576MUXOpenChannelResponse.vi"("error in (no error)"=w275, "Message Data"=w276, "gRPCid"=w277) -> ()  [unwired: 8 in, 1 out]
          }
          event User Event {
            n155 = event-data() -> ("gRPCid"=w294:T24)  [unwired: 1 in, 4 out]
            n156 = Unbundle By Name(w288) -> ("NI2576Session"=w295:refnum<k15>)
            n157 = call <instrlib>:"niSwitch Disconnect All Channels.vi"("instrument handle"=w295) -> ("error out"=w292:errorcluster)  [unwired: 9 in, 1 out]
            n158 = Unbundle(w292) -> ("code"=w297:i32, "source"=w296:string)  [unwired: 1 out]
            n159 = Bundle(cluster=T2 {"errCode"=0, "errMessage"=""} ("error"), "errCode"=w297, "errMessage"=w296) -> (w289:T2)
            n160 = Bundle(cluster=T21 {"error"={"errCode"=0, "errMessage"=""}} ("measurementservice_NI2576MUXDisconnectAllResponse_Data"), "error"=w289) -> (w293:T21)
            n161 = call "Set measurementservice_NI2576MUXDisconnectAllResponse.vi"("error in (no error)"=w292, "Message Data"=w293, "gRPCid"=w294) -> ()  [unwired: 8 in, 1 out]
          }
          event User Event {
            n162 = event-data() -> ("gRPCid"=w300:T24)  [unwired: 1 in, 4 out]
            n163 = Unbundle By Name(w298) -> ("NI2576Session"=w299:refnum<k15>)
            n164 = call <instrlib>:"niSwitch Close.vi"("instrument handle"=w299) -> ("error out"=w302:errorcluster)  [unwired: 10 in]
            n165 = Unbundle(w302) -> ("code"=w304:i32, "source"=w303:string)  [unwired: 1 out]
            n166 = Bundle(cluster=T2 {"errCode"=0, "errMessage"=""} ("error"), "errCode"=w304, "errMessage"=w303) -> (w305:T2)
            n167 = Bundle(cluster=T22 {"error"={"errCode"=0, "errMessage"=""}} ("measurementservice_NI2576MUXCloseSessionResponse_Data"), "error"=w305) -> (w301:T22)
            n168 = call "Set measurementservice_NI2576MUXCloseSessionResponse.vi"("error in (no error)"=w302, "Message Data"=w301, "gRPCid"=w300) -> ()  [unwired: 8 in, 1 out]
          }
          event User Event {
            n169 = event-data() -> ("gRPCid"=w313:T24)  [unwired: 1 in, 4 out]
            n170 = Unbundle By Name(w308) -> ("NI2576Session"=w314:refnum<k15>)
            n171 = call <instrlib>:"niSwitch Reset.vi"("instrument handle"=w314) -> ("error out"=w311:errorcluster)  [unwired: 9 in, 1 out]
            n172 = Unbundle(w311) -> ("code"=w316:i32, "source"=w315:string)  [unwired: 1 out]
            n173 = Bundle(cluster=T2 {"errCode"=0, "errMessage"=""} ("error"), "errCode"=w316, "errMessage"=w315) -> ()  [unwired: 1 out]
            n174 = Bundle(cluster=T10 {"error"={"errCode"=0, "errMessage"=""}} ("measurementservice_DMMResetResponse_Data")) -> (w312:T10)  [unwired: 1 in]
            n175 = call "Set measurementservice_DMMResetResponse.vi"("error in (no error)"=w311, "Message Data"=w312, "gRPCid"=w313) -> ()  [unwired: 8 in, 1 out]
          }
        }
      }
      n176 = Unregister For Events(event registration refnum=w11, error in=w10) -> (error out=w9:errorcluster)
    }
    frame Error {
    }
  }
  "error out" <- w5
  "gRPC Server out" <- w3
